vi "UHR-Fleezers Control (host) - 10.5.vi"() -> ()   [LabVIEW 2011] (continued)
        n935 = xnode "Read/Write Control"("FPGA VI Reference In"=w1438, "error in"=w1437, "Scan steps"=w1377, "Number of scans"="Number of F/B Scans (AOD)", "Cycles per step"=w1345, "Scan freq.  increment"=w1383, "Scan BD"="Scan BD") -> ("error out"=w1436:errorcluster)  [unwired: 1 out]
        n936 = Multiply(x=w1377, y=w1345) -> (x*y=w1431:u64)
        n937 = Multiply(x=w1431, y=u64 2) -> (x*y=w1353:u64)
        n938 = Multiply(x=w1354, y=w1353) -> (x*y=w1352:dbl)
        "Data points/scan (f/b)" <- w1352
        n939 = Multiply(x=w1352, y="Number of F/B Scans (AOD)") -> (x*y=w1434:dbl)
        "Data points/scans" <- w1434
        n940 = Divide(x=w1434, y=w1388) -> (x/y=→"N sets should be saved":dbl)
        n941 = Multiply(x=w1431, y=w1372) -> (x*y=w1370:dbl)
        "Time/Scan (s) (AOD)" <- w1370
        n942 = Select(t=w1402, s="Scan BD", f=0.0) -> (s? t:f=w1428:dbl)
        n943 = Select(t=0.0, s="Scan BD", f=w1402) -> (s? t:f=w1424:dbl)
        n944 = local read "BD 2 Frequency 2 (MHz)"() -> (w1420:dbl)
        n945 = local read "BD 1 Frequency 2 (MHz)"() -> (w1423:dbl)
        n946 = Add(x=w1424, y=w1395) -> (x+y=w1421:dbl)
        n947 = Add(x=w1389, y=w1428) -> (x+y=w1422:dbl)
        n948 = Multiply(x=w1370, y=2.0) -> (x*y=w1369:dbl)
        n949 = Multiply(x=w1369, y="Number of F/B Scans (AOD)") -> (x*y=w1366:dbl)
        n950 = Divide(x=w1366, y=60.0) -> (x/y=→"Time to Finish All (min)":dbl)
        n951 = Add(x="Trap 2 Bead Size (nm)", y="Trap 1 Bead Size (nm)") -> (x+y=w1410:dbl)
        n952 = Divide(x=w1410, y=2.0) -> (x/y=w1404:dbl)
        n953 = local read "Initial delta (MHz)"() -> (w1407:dbl)
        n954 = Subtract(x=w1421, y=w1420) -> (x-y=w1418:dbl)
        n955 = Subtract(x=w1422, y=w1423) -> (x-y=w1419:dbl)
        n956 = Square(x=w1418) -> (x^2=w1417:dbl)
        n957 = Square(x=w1419) -> (x^2=w1416:dbl)
        n958 = Add(x=w1416, y=w1417) -> (x+y=w1415:dbl)
        n959 = Square Root(x=w1415) -> (sqrt(x)=w1414:dbl)
        "Final delta (MHz)" <- w1414
        n960 = Multiply(x=w1406, y=w1414) -> (x*y=w1413:dbl)
        n961 = Multiply(x=w1407, y=w1406) -> (x*y=w1405:dbl)
        n962 = Subtract(x=w1405, y=w1404) -> (x-y=→"Initial sep (nm)":dbl)
        n963 = Subtract(x=w1413, y=w1404) -> (x-y=→"Final sep (nm)":dbl)
      }
      event "Freq or Amp switch first", "Swap F1 and F2", "Freq switch delay", "Amp switch delay": Value Change {
        n964 = event-data() -> ()  [unwired: 7 out]
        n965 = local read "Freq or Amp switch first"() -> (w1439:bool)
        n966 = local read "Amp switch delay"() -> (w1440:u16)
        n967 = local read "Freq switch delay"() -> (w1442:u16)
        n968 = local read "Swap F1 and F2"() -> (w1441:bool)
        n969 = xnode "Read/Write Control"("FPGA VI Reference In"=w1445, "error in"=w1444, "Freq switch delay"=w1442, "Swap F1 and F2"=w1441, "Amp switch delay"=w1440, "Freq or Amp switch first"=w1439) -> ("error out"=w1443:errorcluster)  [unwired: 1 out]
      }
      event "Scan steps (MCL)", "Number of scans (MCL)", "Scan Range (V)\n(of steps)", "2D or 1D Scan", "N APD Samp/step", "Fast Scan Dir", "Continuous MCL Scanning", "Scan lines (y)": Value Change {
        w1447 = 32767.0 ("y")
        n970 = event-data() -> ()  [unwired: 7 out]
        n971 = Select(t="Scan lines (y)", s="2D or 1D Scan", f="Number of scans (MCL)") -> (s? t:f=w1452:u64)
        n972 = Decrement(x="Scan steps (MCL)") -> (x-1=w1468:u64)
        n973 = Divide(x="Scan Range (V)\n(of steps)", y=w1468) -> (x/y=w1467:dbl)
        "Desired Scan Incr (V)" <- w1467
        n974 = local read "APD Integration Time (s)"() -> (w1460:dbl)
        n975 = Multiply(x=w1467, y=w1447) -> (x*y=w1476:dbl)
        n976 = Divide(x=w1476, y=10.0) -> (x/y=w1466:dbl)
        "Desired incr (int)" <- w1466
        n977 = local read "Update Count (MCL)"() -> (w1472:u32)
        n978 = Round Toward -Infinity(1:w1466) -> (0:w1475:dbl)
        n979 = To Word Integer(number=w1475) -> (16bit integer=w1450:i16)
        "Actual Incr. int (MCL)" <- w1450
        n980 = Multiply(x=w1460, y=40000000.0) -> (x*y=w1473:dbl)
        n981 = Divide(x=w1473, y=w1472) -> (x/y=w1471:dbl)
        n982 = Multiply(x=i16 10, y=w1450) -> (x*y=w1448:i16)
        n983 = Multiply(x="N APD Samp/step", y=w1471) -> (x*y=w1470:dbl)
        "Cycles/step (MCL)" <- w1470
        n984 = Divide(x=w1448, y=w1447) -> (x/y=→"Actual MCL Inc (V)":dbl)
        n985 = Multiply(x="N APD Samp/step", y="Scan steps (MCL)") -> (x*y=w1462:dbl)
        n986 = local read "APD Samples/FIFO Acq."() -> (w1459:dbl)
        n987 = Multiply(x=w1462, y=u64 2) -> (x*y=w1461:dbl)
        "Data points/scan (f+b)" <- w1461
        n988 = Multiply(x=w1461, y=w1452) -> (x*y=w1479:dbl)
        "Data points/scans (MCL)" <- w1479
        n989 = Multiply(x=w1460, y=w1461) -> (x*y=w1453:dbl)
        "Time/f+b scan (s) (MCL)" <- w1453
        n990 = Divide(x=w1479, y=w1459) -> (x/y=→"N sets should be saved (MCL)":dbl)
        n991 = Multiply(x=w1453, y=w1452) -> (x*y=→"Total Time (s)":dbl)
        n992 = Not(x="Fast Scan Dir") -> (.not. x?=w1457:bool)
        n993 = xnode "Read/Write Control"("FPGA VI Reference In"=w1483, "error in"=w1482, "Scan steps (MCL)"="Scan steps (MCL)", "Number of scans (MCL)"=w1452, "Cycles per step (MCL)"=w1470, "Scan freq.  increment (MCL)"=w1450, "1D or 2D Scan?"="2D or 1D Scan", "MCL Scan Axis"=w1457, "Cont. Scan (MCL)"="Continuous MCL Scanning") -> ("error out"=w1481:errorcluster)  [unwired: 1 out]
      }
      event "Read Cal": Value Change {
        w1485 = 1000.0 ("y")
        n994 = event-data() -> ()  [unwired: 7 out]
        n995 = local read "Save file name"() -> (w1510:path)
        n996 = local write "Read Cal"(FALSE ("Read Cal")) -> ()
        n997 = Strip Path(path=w1510) -> (stripped path=w1509:path)  [unwired: 1 out]
        n998 = Path To String(path=w1509) -> (string=w1508:string)
        n999 = Concatenate Strings(w1508, "\\current.cal" ("string")) -> (w1506:string)
        n1000 = String To Path(string=w1506) -> (path=w1505:path)
        n1001 = Open/Create/Replace File(file path (use dialog)=w1505, operation (0:open)=T25."open", access (0:read/write)=enum16{"read/write", "read-only", "write-only"}."read-only") -> (refnum out=w1513:refnum<file>, error out=w1499:errorcluster)  [unwired: 1 in, 3 out]
        n1002 = Deny Access(4:w1499, 7:w1513) -> (0:w1498:errorcluster, 3:w1504:refnum<file>)  [unwired: 1 out]
        n1003 = Read from Binary File(5:0.0, 8:w1498, 9:T24."big-endian, network order" ("byte order (0:big-endian, network order)"), 10:-1 ("count (1)"), 11:w1504) -> (0:w1497:errorcluster, 2:w1495:dbl[], 3:w1500:refnum<file>)  [unwired: 2 out]
        n1004 = Array To Cluster(array=w1495) -> (cluster=w1494:T27)
        n1005 = Unbundle(w1494) -> ("[0]"=w1493:dbl, "[1]"=w1492:dbl, "[2]"=w1491:dbl, "[3]"=w1490:dbl, "[4]"=w1489:dbl, "[5]"=w1488:dbl)
        n1006 = Close File(refnum=w1500, error in=w1497) -> (error out=→"Read cal error":errorcluster)  [unwired: 1 out]
        n1007 = Multiply(x=w1488, y=w1485) -> (x*y=w1486:dbl)
        n1008 = local write "T2 kappa_x (pN/nm)"(w1490) -> ()
        n1009 = local write "T1 kappa_x (pN/nm)"(w1491) -> ()
        n1010 = local write "T1 alpha_x (nm/V)"(w1493) -> ()
        n1011 = local write "T2 alpha_x (nm/V)"(w1492) -> ()
        n1012 = Multiply(x=w1489, y=w1485) -> (x*y=w1487:dbl)
        n1013 = local write "T1 offset_x (mV)"(w1487) -> ()
        n1014 = local write "T2 offset_x (mV)"(w1486) -> ()
      }
      event "Abort MCL Scan": Value Change {
        n1015 = event-data() -> ()  [unwired: 7 out]
        n1016 = local write "MCL Scanning"(FALSE ("MCL Scanning")) -> ()
        n1017 = xnode "Read/Write Control"("FPGA VI Reference In"=w1518, "error in"=w1517, "Abort scan (MCL)"="Abort MCL Scan") -> ("error out"=w1516:errorcluster)  [unwired: 1 out]
      }
      event "Update Count (MCL)": Value Change {
        n1018 = event-data() -> ()  [unwired: 7 out]
        n1019 = xnode "Read/Write Control"("FPGA VI Reference In"=w1522, "error in"=w1521, "MCL count"="Update Count (MCL)") -> ("error out"=w1520:errorcluster)  [unwired: 1 out]
      }
      event "Phase adjust (MCL)", "+ phase (MCL)", "- phase (MCL)": Value Change {
        n1020 = event-data() -> ()  [unwired: 7 out]
        n1021 = Negate(x="Phase adjust (MCL)") -> (-x=w1531:i16)
        n1022 = Select(t=w1531, s="- phase (MCL)", f="Phase adjust (MCL)") -> (s? t:f=w1529:i16)
        n1023 = Or(x="- phase (MCL)", y="+ phase (MCL)") -> (x .or. y?=w1524:bool)
        n1024 = xnode "Read/Write Control"("FPGA VI Reference In"=w1533, "error in"=w1532, "Phase count adjustment (MCL)"=w1529) -> ("FPGA VI Reference Out"=w1525:T19, "error out"=w1526:errorcluster)
        n1025 = xnode "Read/Write Control"("FPGA VI Reference In"=w1525, "error in"=w1526, "+ phase (MCL)"=w1524) -> ("error out"=w1523:errorcluster)  [unwired: 1 out]
      }
      event "Abort AOD Scan": Value Change {
        n1026 = event-data() -> ()  [unwired: 7 out]
        n1027 = xnode "Read/Write Control"("FPGA VI Reference In"=w1537, "error in"=w1536, "Abort scan"="Abort AOD Scan") -> ("error out"=w1535:errorcluster)  [unwired: 1 out]
      }
      event "Continuous AOD Scanning": Value Change {
        n1028 = event-data() -> ()  [unwired: 7 out]
        n1029 = xnode "Read/Write Control"("FPGA VI Reference In"=w1541, "error in"=w1540, "Cont. Scan"="Continuous AOD Scanning") -> ("error out"=w1539:errorcluster)  [unwired: 1 out]
      }
      event "Index": Value Change {
        n1030 = event-data() -> ()  [unwired: 7 out]
        n1031 = call "Create new save file.vi"("Insert"="", "Ext"=".dat" ("string"), "Index In"="Index") -> ("Path Out"=→"Save file name":path, "Index Out"=w1542:dbl)
        "Save index" <- w1542
        n1032 = local write "Index"(w1542) -> ()
      }
      event "AO1", "AO2": Value Change {
        w1557 = 10.0 ("y")
        w1556 = 32767.0 ("y")
        n1033 = event-data() -> ()  [unwired: 7 out]
        n1034 = local read "AO2"() -> (w1555:dbl)
        n1035 = local read "AO1"() -> (w1552:dbl)
        n1036 = Multiply(x=w1552, y=w1556) -> (x*y=w1551:dbl)
        n1037 = Multiply(x=w1555, y=w1556) -> (x*y=w1554:dbl)
        n1038 = Divide(x=w1551, y=w1557) -> (x/y=w1550:dbl)
        n1039 = Divide(x=w1554, y=w1557) -> (x/y=w1553:dbl)
        n1040 = To Word Integer(number=w1550) -> (16bit integer=w1558:i16)
        n1041 = To Word Integer(number=w1553) -> (16bit integer=w1559:i16)
        n1042 = xnode "Read/Write Control"("FPGA VI Reference In"=w1549, "error in"=w1548, "AO1"=w1558, "AO2"=w1559) -> ("error out"=w1547:errorcluster)  [unwired: 1 out]
      }
      event "Inject Pump 1": Value Change {
        n1043 = local read "Chemyx Syringe Pump Serial Port"() -> (w1560:refnum<visa-resource-name>)
        n1044 = event-data() -> ()  [unwired: 7 out]
        n1045 = local read "Pump write delay (ms)"() -> (w1561:dbl)
        n1046 = case shown="False" "Inject Pump 1" {
          tunnel: w1561 -> [w1568 w1582]
          tunnel: w1560 -> [w1565 w1581]
          frame False {
            n1047 = flat-sequence {
              tunnel: w1565 -> [w1569]
              tunnel: [w1569] -> w1566
              tunnel: w1568 -> [_]
              tunnel: [w1572] -> w1567
              tunnel: w1566 -> [w1572]
              tunnel: w1567 -> [w1573]
              tunnel: [w1573] -> w1563
              tunnel: [w1575] -> w1564
              tunnel: w1563 -> [w1575]
              tunnel: w1564 -> [w1577]
              frame #0 {
                n1048 = call "Write to pump.vi"("string"="enter pump1", "VISA resource name"=w1569) -> ()  [unwired: 1 out]
              }
              frame #1 {
                n1049 = Wait (ms)(milliseconds to wait="Pump pause delay (ms)") -> ()  [unwired: 1 out]
              }
              frame #2 {
                n1050 = call "Write to pump.vi"("string"="stop", "VISA resource name"=w1573) -> ()  [unwired: 1 out]
              }
              frame #3 {
                n1051 = Wait (ms)(milliseconds to wait=u32 500) -> ()  [unwired: 1 out]
              }
              frame #4 {
                n1052 = call "Write to pump.vi"("string"="stop", "VISA resource name"=w1577) -> ()  [unwired: 1 out]
              }
            }
          }
          frame True {
            n1053 = flat-sequence {
              tunnel: w1581 -> [w1591]
              tunnel: w1582 -> [w1586]
              tunnel: w1582 -> [w1593]
              tunnel: w1581 -> [w1594]
              tunnel: [w1594] -> w1579
              tunnel: [w1596] -> w1580
              tunnel: w1579 -> [w1596]
              tunnel: w1580 -> [w1598]
              frame #0 {
                n1054 = local read "All Pump Parameters"() -> (w1585:T1)
                n1055 = Unbundle By Name(w1585) -> ("Pump 1"=w1592:T28)
                n1056 = call "Set pump parameters.vi"("Pump write delay (ms)"=w1586, "Volume (uL)"="Ch 1 Inject Volume (uL)", "Rate (uL/h)"="Ch 1 Inject Rate (ul/h)", "Units"=4.0, "Pump #"=1.0, "Pump Parameters In"=w1592, "VISA resource name"=w1591) -> ("Pump Parameters Out"=w1584:T28)  [unwired: 3 in]
                n1057 = Bundle By Name(cluster=w1585, "Pump 1"=w1584) -> (w1583:T1)
                n1058 = local write "All Pump Parameters"(w1583) -> ()
              }
              frame #1 {
                n1059 = Wait (ms)(milliseconds to wait=w1593) -> ()  [unwired: 1 out]
              }
              frame #2 {
                n1060 = call "Write to pump.vi"("string"="start", "VISA resource name"=w1594) -> ()  [unwired: 1 out]
              }
              frame #3 {
                n1061 = Wait (ms)(milliseconds to wait=u32 500) -> ()  [unwired: 1 out]
              }
              frame #4 {
                n1062 = call "Write to pump.vi"("string"="start", "VISA resource name"=w1598) -> ()  [unwired: 1 out]
              }
            }
          }
        }
      }
      event "Inject Pump 3": Value Change {
        n1063 = event-data() -> ()  [unwired: 7 out]
        n1064 = local read "Pump write delay (ms)"() -> (w1601:dbl)
        n1065 = case shown="False" "Inject Pump 3" {
          tunnel: w1601 -> [w1608 w1622]
          tunnel: "Chemyx Syringe Pump Serial Port" -> [w1605 w1621]
          frame False {
            n1066 = flat-sequence {
              tunnel: w1605 -> [w1609]
              tunnel: [w1609] -> w1606
              tunnel: w1608 -> [_]
              tunnel: [w1612] -> w1607
              tunnel: w1606 -> [w1612]
              tunnel: w1607 -> [w1613]
              tunnel: [w1613] -> w1603
              tunnel: [w1615] -> w1604
              tunnel: w1603 -> [w1615]
              tunnel: w1604 -> [w1617]
              frame #0 {
                n1067 = call "Write to pump.vi"("string"="enter pump3", "VISA resource name"=w1609) -> ()  [unwired: 1 out]
              }
              frame #1 {
                n1068 = local read "Pump pause delay (ms)"() -> (w1611:u32)
                n1069 = Wait (ms)(milliseconds to wait=w1611) -> ()  [unwired: 1 out]
              }
              frame #2 {
                n1070 = call "Write to pump.vi"("string"="stop", "VISA resource name"=w1613) -> ()  [unwired: 1 out]
              }
              frame #3 {
                n1071 = Wait (ms)(milliseconds to wait=u32 0) -> ()  [unwired: 1 out]
              }
              frame #4 {
                n1072 = call "Write to pump.vi"("string"="stop", "VISA resource name"=w1617) -> ()  [unwired: 1 out]
              }
            }
          }
          frame True {
            n1073 = flat-sequence {
              tunnel: w1621 -> [w1631]
              tunnel: w1622 -> [w1626]
              tunnel: w1622 -> [w1633]
              tunnel: w1621 -> [w1634]
              tunnel: [w1634] -> w1619
              tunnel: [w1637] -> w1620
              tunnel: w1619 -> [w1637]
              tunnel: w1620 -> [w1638]
              frame #0 {
                n1074 = local read "All Pump Parameters"() -> (w1625:T1)
                n1075 = Unbundle By Name(w1625) -> ("Pump 3"=w1632:T28)
                n1076 = call "Set pump parameters.vi"("Pump write delay (ms)"=w1626, "Volume (uL)"="Ch 3 Inject Volume (uL)", "Rate (uL/h)"="Ch 3 Inject Rate (ul/h)", "Units"=4.0, "Pump #"=3.0, "Pump Parameters In"=w1632, "VISA resource name"=w1631) -> ("Pump Parameters Out"=w1624:T28)  [unwired: 3 in]
                n1077 = Bundle By Name(cluster=w1625, "Pump 3"=w1624) -> (w1623:T1)
                n1078 = local write "All Pump Parameters"(w1623) -> ()
              }
              frame #1 {
                n1079 = Wait (ms)(milliseconds to wait=w1633) -> ()  [unwired: 1 out]
              }
              frame #2 {
                n1080 = call "Write to pump.vi"("string"="start", "VISA resource name"=w1634) -> ()  [unwired: 1 out]
              }
              frame #3 {
                n1081 = Wait (ms)(milliseconds to wait=u32 500) -> ()  [unwired: 1 out]
              }
              frame #4 {
                n1082 = call "Write to pump.vi"("string"="start", "VISA resource name"=w1638) -> ()  [unwired: 1 out]
              }
            }
          }
        }
      }
      event "Inject Pump 2": Value Change {
        n1083 = event-data() -> ()  [unwired: 7 out]
        n1084 = local read "Pump write delay (ms)"() -> (w1642:dbl)
        n1085 = flat-sequence {
          tunnel: w1640 -> [w1655]
          tunnel: w1642 -> [w1651]
          tunnel: "Inject Pump 2" -> [_]
          tunnel: w1642 -> [w1657]
          tunnel: w1640 -> [w1658]
          frame #0 {
            n1086 = local read "All Pump Parameters"() -> (w1650:T1)
            n1087 = Multiply(x=60.0, y="Flush Center Ch Rate (ul/m)") -> (x*y=w1647:dbl)
            n1088 = Unbundle By Name(w1650) -> ("Pump 2"=w1656:T28)
            n1089 = call "Set pump parameters.vi"("Pump write delay (ms)"=w1651, "Volume (uL)"="Flush Center Ch Volume (uL)", "Rate (uL/h)"=w1647, "Units"=3.0, "Pump #"=2.0, "Pump Parameters In"=w1656, "VISA resource name"=w1655) -> ("Pump Parameters Out"=w1649:T28)  [unwired: 3 in]
            n1090 = Bundle By Name(cluster=w1650, "Pump 2"=w1649) -> (w1648:T1)
            n1091 = local write "All Pump Parameters"(w1648) -> ()
            n1092 = Add(x="Flush Center Ch Volume (uL)", y="Total Volume\nFlushed (uL)") -> (x+y=w1644:dbl)
            n1093 = local write "Total Volume\nFlushed (uL)"(w1644) -> ()
          }
          frame #1 {
            n1094 = Wait (ms)(milliseconds to wait=w1657) -> ()  [unwired: 1 out]
          }
          frame #2 {
            n1095 = call "Write to pump.vi"("string"="start", "VISA resource name"=w1658) -> ()  [unwired: 1 out]
          }
        }
        n1096 = local read "Chemyx Syringe Pump Serial Port"() -> (w1640:refnum<visa-resource-name>)
      }
      event "Sample Channel\nFlow": Value Change {
        n1097 = event-data() -> ()  [unwired: 7 out]
        n1098 = case shown="True" "Sample Channel\nFlow" {
          tunnel: w1662 -> [w1668 w1670]
          tunnel: [w1668 w1669] -> w1661
          frame False {
          }
          frame True {
            n1099 = Number To Decimal String(number="Flow rate (uL/h)") -> (decimal integer string=w1675:string)  [unwired: 1 in]
            n1100 = Concatenate Strings("irate  " ("string"), w1675, " u/h" ("string"), "\r") -> (w1673:string)
            n1101 = VISA Write(VISA resource name=w1670, write buffer=w1673) -> (VISA resource name out=w1669:refnum<visa-resource-name>)  [unwired: 1 in, 2 out]
          }
        }
        n1102 = Select(t="run" ("string"), s="Sample Channel\nFlow", f="stop" ("string")) -> (s? t:f=w1663:string)
        n1103 = Concatenate Strings(w1663, "\r") -> (w1666:string)
        n1104 = VISA Write(VISA resource name=w1661, write buffer=w1666) -> ()  [unwired: 1 in, 3 out]
      }
      event "Flow rate (uL/h)": Value Change {
        n1105 = event-data() -> ()  [unwired: 7 out]
        n1106 = local read "Flow rate (uL/h)"() -> (w1679:dbl)
        n1107 = Number To Decimal String(number=w1679) -> (decimal integer string=w1682:string)  [unwired: 1 in]
        n1108 = Concatenate Strings("irate  " ("string"), w1682, " u/h" ("string"), "\r") -> (w1681:string)
        n1109 = VISA Write(VISA resource name=w1677, write buffer=w1681) -> ()  [unwired: 1 in, 3 out]
      }
      event "Flush Sample": Value Change {
        n1110 = event-data() -> ()  [unwired: 7 out]
        n1111 = Number To Decimal String(number="Flush rate (uL/m)") -> (decimal integer string=w1701:string)  [unwired: 1 in]
        n1112 = Concatenate Strings("irate  " ("string"), w1701, " u/m" ("string"), "\r") -> (w1703:string)
        n1113 = VISA Write(VISA resource name=w1705, write buffer=w1703) -> (VISA resource name out=w1699:refnum<visa-resource-name>)  [unwired: 1 in, 2 out]
        n1114 = Number To Decimal String(number="Volume (uL)") -> (decimal integer string=w1688:string)  [unwired: 1 in]
        n1115 = Concatenate Strings("tvolume  " ("string"), w1688, " u" ("string"), "\r") -> (w1686:string)
        n1116 = VISA Write(VISA resource name=w1699, write buffer=w1686) -> (VISA resource name out=w1685:refnum<visa-resource-name>)  [unwired: 1 in, 2 out]
        n1117 = Concatenate Strings("cvolume" ("string"), "\r") -> (w1684:string)
        n1118 = VISA Write(VISA resource name=w1685, write buffer=w1684) -> (VISA resource name out=w1697:refnum<visa-resource-name>)  [unwired: 1 in, 2 out]
        n1119 = Concatenate Strings("run" ("string"), "\r") -> (w1695:string)
        n1120 = VISA Write(VISA resource name=w1697, write buffer=w1695) -> ()  [unwired: 1 in, 3 out]
      }
      event "Clear Volume": Value Change {
        n1121 = event-data() -> ()  [unwired: 7 out]
        n1122 = Concatenate Strings("cvolume" ("string"), "\r") -> (w1708:string)
        n1123 = VISA Write(VISA resource name=w1707, write buffer=w1708) -> ()  [unwired: 1 in, 3 out]
      }
      event "Flip Green Filter": Value Change {
        n1124 = event-data() -> ()  [unwired: 7 out]
        n1125 = Not(x="Flip Green Filter") -> (.not. x?=w1712:bool)
        n1126 = local write "Flip Green Filter"(w1712) -> ()
        n1127 = flat-sequence {
          tunnel: w1720 -> [w1725]
          tunnel: w1719 -> [w1724]
          tunnel: [w1722] -> w1717
          tunnel: [w1721] -> w1716
          tunnel: [w1727] -> w1715
          tunnel: w1717 -> [w1727]
          tunnel: [w1726] -> w1714
          tunnel: w1716 -> [w1726]
          tunnel: w1715 -> [w1731]
          tunnel: w1714 -> [w1730]
          tunnel: [w1729] -> w1718
          frame #0 {
            n1128 = xnode "Read/Write Control"("FPGA VI Reference In"=w1725, "error in"=w1724, "Green Filter Flipper"=TRUE) -> ("FPGA VI Reference Out"=w1722:T19, "error out"=w1721:errorcluster)
          }
          frame #1 {
            n1129 = Wait (ms)(milliseconds to wait=u32 100) -> ()  [unwired: 1 out]
          }
          frame #2 {
            n1130 = xnode "Read/Write Control"("FPGA VI Reference In"=w1731, "error in"=w1730, "Green Filter Flipper"=FALSE) -> ("error out"=w1729:errorcluster)  [unwired: 1 out]
          }
        }
      }
      event "Pump 1 contents", "Pump 3 contents": Value Change {
        n1131 = event-data() -> ()  [unwired: 7 out]
        n1132 = local read "Pump 1 contents"() -> (→"Pump 1 cont disp":string)
        n1133 = local read "Pump 3 contents"() -> (→"Pump 3 cont disp":string)
      }
      event "Reset Trap Pos. FB": Value Change {
        n1134 = event-data() -> ()  [unwired: 7 out]
        n1135 = xnode "Read/Write Control"("FPGA VI Reference In"=w1737, "error in"=w1736, "Trap Pos. FB Reset"="Reset Trap Pos. FB") -> ()  [unwired: 2 out]
      }
      event "Rem fb disp offset": Value Change {
        n1136 = event-data() -> ()  [unwired: 7 out]
        n1137 = local write "Rem fb disp offset"(FALSE ("Rem fb disp offset")) -> ()
        n1138 = local read "Mean T1 Position (nm)"() -> (w1739:dbl)
        n1139 = local read "FB Trap Pos Offset"() -> (w1740:dbl)
        n1140 = Subtract(x=w1740, y=w1739) -> (x-y=w1738:dbl)
        n1141 = local write "FB Trap Pos Offset"(w1738) -> ()
      }
      event "Threshold (nm)": Value Change {
        n1142 = event-data() -> ()  [unwired: 7 out]
        n1143 = flat-sequence {
          tunnel: w1744 -> [w1752]
          tunnel: w1743 -> [w1751]
          tunnel: [w1745] -> w1742
          tunnel: w1742 -> [w1758]
          frame #0 {
            n1144 = xnode "Read/Write Control"("FPGA VI Reference In"=w1752, "error in"=w1751) -> ("FPGA VI Reference Out"=w1748:T19, "error out"=w1747:errorcluster, "FPGA TTrig Thresh"=w1749:i64)
            n1145 = local read "Threshold stored (nm)"() -> (w1757:dbl)
            n1146 = local read "Threshold (nm)"() -> (w1745:dbl)
            n1147 = local read "AOM X Cal (nm/MHz)"() -> (w1755:dbl)
            n1148 = Subtract(x=w1745, y=w1757) -> (x-y=w1756:dbl)
            n1149 = Divide(x=w1756, y=w1755) -> (x/y=w1753:dbl)
            n1150 = call "IR AOM freq to word.vi"("Frequency In (MHz)"=w1753) -> ("Frequency Word Out (double)"=w1754:dbl)
            n1151 = To Quad Integer(1:w1754) -> (0:w1750:i64)
            n1152 = Add(x=w1749, y=w1750) -> (x+y=w1746:i64)
            n1153 = xnode "Read/Write Control"("FPGA VI Reference In"=w1748, "error in"=w1747, "FPGA TTrig Thresh"=w1746) -> ()  [unwired: 2 out]
          }
          frame #1 {
            "Threshold stored (nm)" <- w1758
          }
        }
      }
      event "FB Trig Integrate": Value Change {
        n1154 = event-data() -> ()  [unwired: 7 out]
        n1155 = local read "FB Trig Integrate"() -> (w1760:u32)
        n1156 = xnode "Read/Write Control"("FPGA VI Reference In"=w1762, "error in"=w1761, "FB Trig Integrate"=w1760) -> ("error out"=w1759:errorcluster)  [unwired: 1 out]
      }
      event "11": Value Change {
        n1157 = event-data() -> ()  [unwired: 7 out]
        n1158 = local read "11"() -> (w1763:bool)
        n1159 = case shown="True" w1763 {
          frame False {
          }
          frame True {
            n1160 = local read "Messages"() -> (w1765:string)
            n1161 = call "Update messages.vi"("Message to add"="You kicked it up to 11!", "Old message string"=w1765) -> ("New message string"=w1766:string)
            n1162 = call <vilib>:"Beep.vi"() -> ()  [unwired: 12 in]
            n1163 = local write "Messages"(w1766) -> ()
          }
        }
      }
      event "Trap Pos. FB ON": Value Change {
        n1164 = event-data() -> ()  [unwired: 7 out]
        n1165 = xnode "Read/Write Control"("FPGA VI Reference In"=w1769, "error in"=w1768, "Force feedback"="Trap Pos. FB ON") -> ()  [unwired: 2 out]
      }
      event "Remove Action Offset": Value Change {
        n1166 = event-data() -> ()  [unwired: 7 out]
        n1167 = local write "Remove Action Offset"(FALSE ("Remove Action Offset")) -> ()
        n1168 = local read "Trap Pos. FB Mult Factor"() -> (w1774:i64)
        n1169 = local read "Trap Pos FB Action"() -> (w1772:i64)
        n1170 = local read "Trap Pos. FB Offset Factor"() -> (w1770:i64)
        n1171 = Multiply(x=w1774, y=w1772) -> (x*y=w1773:i64)
        n1172 = Add(x=w1773, y=w1770) -> (x+y=w1771:i64)
        n1173 = local write "Trap Pos. FB Offset Factor"(w1771) -> ()
        n1174 = xnode "Read/Write Control"("FPGA VI Reference In"=w1777, "error in"=w1776, "Trap Pos. FB Offset Factor"=w1771) -> ()  [unwired: 2 out]
      }
      event "Remove Unwinding Offset": Value Change {
        n1175 = event-data() -> ()  [unwired: 7 out]
        n1176 = local write "Remove Unwinding Offset"(FALSE ("Remove Action Offset")) -> ()
        n1177 = local read "Trap Pos. FB Mult Factor"() -> (w1789:i64)
        n1178 = local read "Trap Pos FB Action"() -> (w1787:i64)
        n1179 = local read "Trap Pos. FB Offset Factor"() -> (w1786:i64)
        n1180 = Multiply(x=w1789, y=w1787) -> (x*y=w1788:i64)
        n1181 = local read "Trap Pos. FB Mult Factor"() -> (w1785:i64)
        n1182 = Add(x=w1788, y=w1786) -> (x+y=w1779:i64)
        n1183 = Multiply(x=32768, y="factor") -> (x*y=w1782:dbl)
        n1184 = Multiply(x=w1782, y=w1785) -> (x*y=w1784:dbl)
        n1185 = Subtract(x=w1779, y=w1784) -> (x-y=w1783:dbl)
        n1186 = To Quad Integer(1:w1783) -> (0:w1778:i64)
        n1187 = xnode "Read/Write Control"("FPGA VI Reference In"=w1792, "error in"=w1791, "Trap Pos. FB Offset Factor"=w1778) -> ()  [unwired: 2 out]
        n1188 = local write "Trap Pos. FB Offset Factor"(w1778) -> ()
      }
      event "Trap Pos. FB Range", "Trap Pos. FB Gains", "Trap Pos. FB Mult Factor", "Trap Pos. FB Offset Factor", "Trap Pos FB Negate Action", "Trap Pos FB Monitor\nT1 or T2", "Differential FB?", "Negate Diff?": Value Change {
        n1189 = event-data() -> ()  [unwired: 7 out]
        n1190 = local read "Negate Diff?"() -> (w1793:bool)
        n1191 = xnode "Read/Write Control"("FPGA VI Reference In"=w1803, "error in"=w1802, "Trap Pos. FB Range"="Trap Pos. FB Range", "Trap Pos. FB Gains"="Trap Pos. FB Gains", "Trap Pos. FB Mult Factor"="Trap Pos. FB Mult Factor", "Trap Pos. FB Offset Factor"="Trap Pos. FB Offset Factor", "Trap Pos FB Negate Action"="Trap Pos FB Negate Action", "Trap Pos FB Monitor T1 or T2"="Trap Pos FB Monitor\nT1 or T2", "AI1 X Scale"="Trap Pos. AI1 X Pre-scale", "Negate Diff?"=w1793, "Diff FB Measurement?"="Differential FB?") -> ()  [unwired: 2 out]
      }
      event "Trap Pos FB SP": Value Change {
        n1192 = event-data() -> ()  [unwired: 7 out]
        n1193 = xnode "Read/Write Control"("FPGA VI Reference In"=w1806, "error in"=w1805, "Trap Pos. FB SP"="Trap Pos FB SP") -> ()  [unwired: 2 out]
      }
      event "Set Reading to\nSetpoint": Value Change {
        # "This is the actual PID input signal"
        n1194 = event-data() -> ()  [unwired: 7 out]
        n1195 = local write "Set Reading to\nSetpoint"(FALSE ("Set SP to Reading")) -> ()
        n1196 = xnode "Read/Write Control"("FPGA VI Reference In"=w1811, "error in"=w1810) -> ("FPGA VI Reference Out"=w1809:T19, "error out"=w1808:errorcluster, "Trap Pos FB Int-Norm Signal"=w1807:fxp<+/-,16,1>)
        n1197 = local read "Differential FB?"() -> (w1812:bool)
        n1198 = case shown="False" w1812 {
          tunnel: [w1817 w1824] -> w1814
          tunnel: w1807 -> [w1815 w1824]
          frame False {
            n1199 = local read "Trap Pos FB Monitor\nT1 or T2"() -> (w1820:bool)
            n1200 = local read "Trap X AI1 (DMA)"() -> (w1823:T13)
            n1201 = Unbundle By Name(w1823) -> ("Set 1"=w1822:fxp<+/-,16,1>, "Set 2"=w1821:fxp<+/-,16,1>)
            n1202 = Select(t=w1822, s=w1820, f=w1821) -> (s? t:f=w1819:fxp<+/-,16,1>)
            n1203 = Not(x="Set SP Using...") -> (.not. x?=w1816:bool)
            n1204 = Select(t=w1815, s=w1816, f=w1819) -> (s? t:f=w1817:fxp<+/-,16,1>)
          }
          frame True {
          }
        }
        n1205 = xnode "Read/Write Control"("FPGA VI Reference In"=w1809, "error in"=w1808, "Trap Pos. FB SP"=w1814) -> ()  [unwired: 2 out]
        n1206 = local write "Trap Pos FB SP"(w1814) -> ()
      }
      event "Trap Pos. FB Out Scale 2^n": Value Change {
        n1207 = event-data() -> ()  [unwired: 7 out]
        n1208 = Scale By Power Of 2(n="Trap Pos. FB Out Scale 2^n", x=ext 1.0) -> (x*2^n=w1825:ext)
        n1209 = property on="Trap Pos. FB Mult Factor" class="DigNum (strict)"("Val(Sgnl)"=w1825) -> ()  [unwired: 2 in, 2 out]
      }
      event "Trap Pos FB Int Count": Value Change {
        n1210 = event-data() -> ()  [unwired: 7 out]
        n1211 = xnode "Read/Write Control"("FPGA VI Reference In"=w1830, "error in"=w1829, "Trap Pos FB Int Count"="Trap Pos FB Int Count") -> ()  [unwired: 2 out]
      }
    }
    "error out 2" <- w950
    n1212 = node-c288() -> ()  [unwired: 2 out]
  }
  n1213 = disable-structure shown="Disabled" {
    disable-tunnel: [w1832 _] -> w220
    disable-tunnel: w40 -> [w1831 _]
    frame Disabled {
      n1214 = node-c288() -> (w1834:T21)  [unwired: 4 out]
      n1215 = timed-loop "Rough control of MCL mirror stage (debugging)" {
        tunnel: w1831 -> [w1837]
        tunnel: [w1836] -> w1832
        timing: w1834 -> [_]
        timing-out: [_] -> w1833
        stop <- w1836 stop-if-true
        n1216 = node-c288() -> ()  [unwired: 2 out]
        n1217 = case shown="1" "MCL Mode" {
          tunnel: w1837 -> [_ w1840 w1887]
          frame 0, Default {
          }
          frame 1 {
            n1218 = node-c288() -> (w1842:T21)  [unwired: 4 out]
            n1219 = timed-loop "Oscillate MCL mirror" {
              timing: w1842 -> [_]
              timing-out: [_] -> w1841
              tunnel: w1840 -> [w1881]
              i -> [w1880]
              stop <- w1843 stop-if-true
              n1220 = node-c288() -> (w1879:i64)  [unwired: 1 out]
              n1221 = Multiply(x="AO1", y=32767.0) -> (x*y=w1875:dbl)
              n1222 = Multiply(x="AO2", y=32767.0) -> (x*y=w1870:dbl)
              n1223 = Divide(x=w1875, y=10.0) -> (x/y=w1876:dbl)
              n1224 = Divide(x=w1870, y=10.0) -> (x/y=w1871:dbl)
              n1225 = To Word Integer(number=w1876) -> (16bit integer=w1868:i16)
              n1226 = To Word Integer(number=w1871) -> (16bit integer=w1867:i16)
              n1227 = Divide(x=w1879, y=i64 1000) -> (x/y=w1850:dbl)
              n1228 = Multiply(x=w1850, y=w1880) -> (x*y=w1861:dbl)
              n1229 = Multiply(x="Osc. freq. (Hz) 2", y=6.283185307179586) -> (x*y=w1862:dbl)
              n1230 = Multiply(x=w1862, y=w1861) -> (x*y=w1860:dbl)
              n1231 = Sine(x=w1860) -> (sin(x)=w1859:dbl)
              n1232 = Multiply(x=w1859, y="Osc. amp. (V)") -> (x*y=w1857:dbl)
              n1233 = Add(x=w1857, y="Osc. center (V)") -> (x+y=w1855:dbl)
              n1234 = Divide(x=w1855, y=10.0) -> (x/y=w1853:dbl)
              n1235 = Multiply(x=w1853, y=32767.0) -> (x*y=w1848:dbl)
              n1236 = Select(t=w1848, s="Scan axis", f=w1868) -> (s? t:f=w1866:dbl)
              n1237 = Select(t=w1867, s="Scan axis", f=w1848) -> (s? t:f=w1865:dbl)
              n1238 = local read "MCL Mode"() -> (w1847:u16)
              n1239 = Not Equal?(x=w1847, y=u16 1) -> (x != y?=w1844:bool)
              n1240 = local read "Stop All"() -> (w1845:bool)
              n1241 = xnode "Read/Write Control"("FPGA VI Reference In"=w1881, "AO1"=w1866, "AO2"=w1865) -> ()  [unwired: 1 in, 2 out]
              n1242 = Compound Arithmetic op=OR(w1845, w1844) -> (w1843:bool)
              n1243 = node-c288() -> ()  [unwired: 2 out]
            }
            n1244 = node-c288(w1841) -> ()  [unwired: 1 out]
          }
          frame 2 {
            n1245 = case shown="True" "Start Scan" {
              tunnel: w1887 -> [_ w1899]
              frame False {
              }
              frame True {
                n1246 = Subtract(x="End (V)", y="Begin (V)") -> (x-y=w1895:dbl)
                n1247 = Decrement(x="N Points") -> (x-1=w1894:dbl)
                n1248 = Divide(x=w1895, y=w1894) -> (x/y=w1892:dbl)
                n1249 = for {
                  N: "N Points" -> [_]
                  tunnel: "Begin (V)" -> [w1912]
                  tunnel: w1899 -> [w1904]
                  tunnel: [w1903] -> w1898 mode=indexing
                  tunnel: w1892 -> [w1902]
                  tunnel: [w1900] -> w1891 mode=indexing
                  i -> [w1911]
                  n1250 = Multiply(x=w1902, y=w1911) -> (x*y=w1910:dbl)
                  n1251 = Add(x=w1912, y=w1910) -> (x+y=w1907:dbl)
                  n1252 = local read "Scan axis"() -> (w1901:bool)
                  n1253 = local read "AO1"() -> (w1909:dbl)
                  n1254 = local read "AO2"() -> (w1908:dbl)
                  n1255 = Select(t=w1907, s=w1901, f=w1909) -> (s? t:f=w1906:dbl)
                  n1256 = Select(t=w1908, s=w1901, f=w1907) -> (s? t:f=w1905:dbl)
                  n1257 = flat-sequence {
                    tunnel: w1906 -> [w1916]
                    tunnel: w1905 -> [w1915]
                    tunnel: w1904 -> [w1913]
                    tunnel: [w1926] -> w1903
                    tunnel: [w1925] -> w1900
                    frame #0 {
                      w1919 = 10.0 ("y")
                      w1914 = 32767.0 ("y")
                      n1258 = Multiply(x=w1916, y=w1914) -> (x*y=w1922:dbl)
                      n1259 = Multiply(x=w1915, y=w1914) -> (x*y=w1920:dbl)
                      n1260 = Divide(x=w1922, y=w1919) -> (x/y=w1923:dbl)
                      n1261 = Divide(x=w1920, y=w1919) -> (x/y=w1921:dbl)
                      n1262 = To Word Integer(number=w1923) -> (16bit integer=w1917:i16)
                      n1263 = To Word Integer(number=w1921) -> (16bit integer=w1918:i16)
                      n1264 = xnode "Read/Write Control"("FPGA VI Reference In"=w1913, "AO1"=w1917, "AO2"=w1918) -> ()  [unwired: 1 in, 2 out]
                    }
                    frame #1 {
                      n1265 = Wait (ms)(milliseconds to wait="DAQ Delay (ms)") -> ()  [unwired: 1 out]
                    }
                    frame #2 {
                      n1266 = local read "Slow mean"() -> (w1926:dbl)
                      n1267 = local read "Sigma"() -> (w1925:dbl)
                    }
                  }
                }
                n1268 = Bundle("Begin (V)"="Begin (V)", w1892, w1898) -> (→"MCL Scan":cluster{"Begin (V)":dbl, dbl, dbl[]})  [unwired: 1 out]
                n1269 = Bundle("Begin (V)"="Begin (V)", w1892, w1891) -> (→"MCL Scan 2":cluster{"Begin (V)":dbl, dbl, dbl[]})  [unwired: 1 out]
              }
            }
          }
        }
        n1270 = local read "Stop All"() -> (w1836:bool)
        n1271 = node-c288() -> ()  [unwired: 2 out]
      }
      n1272 = node-c288(w1833) -> ()  [unwired: 1 out]
    }
    frame Enabled {
    }
  }
  n1273 = node-c288() -> (w84:T21)  [unwired: 4 out]
  n1274 = node-c288(3 ("Processor")) -> (w80:T21)  [unwired: 3 out]
  n1275 = timed-loop "Mouse control: trap position (AOM deflection), set confocal spot from image" {
    tunnel: [w1930] -> w172
    tunnel: w40 -> [w1929]
    timing: w84 -> [_]
    timing-out: [_] -> w83
    stop <- w1930 stop-if-true
    n1276 = node-c288() -> ()  [unwired: 2 out]
    n1277 = event shown="[0] \"Pane\": Mouse Down" {
      selector: _ -> [_ _]
      dyn-events: _ -> [_ _]
      timeout: _ -> [_ _]
      tunnel: w1929 -> [w1933 _]
      event Mouse Down {
        n1278 = event-data() -> ("Time"=w1935:u32, "Coords"=w1934:T7, "Button"=w1936:u16)  [unwired: 6 out]
        n1279 = case shown="1" w1936 {
          tunnel: w1935 -> [_ _ w2039]
          tunnel: w1934 -> [_ w1973 w2037]
          tunnel: w1933 -> [_ _ w2035]
          frame 0, Default {
          }
          frame 1 {
            n1280 = property on="APD 2" class="ImageControl"() -> ("Displayed Image Position"=w1943:cluster{"Left":i32, "Top":i32})  [unwired: 2 in, 2 out]
            n1281 = property on="APD 1" class="ImageControl"() -> ("Displayed Image Position"=w1972:cluster{"Left":i32, "Top":i32})  [unwired: 2 in, 2 out]
            n1282 = property on="Detection Laser X" class="ImageControl"() -> ("Displayed Image Position"=w1969:cluster{"Left":i32, "Top":i32})  [unwired: 2 in, 2 out]
            n1283 = property on="Detection Laser Y" class="ImageControl"() -> ("Displayed Image Position"=w1968:cluster{"Left":i32, "Top":i32})  [unwired: 2 in, 2 out]
            n1284 = property on="APD 2" class="ImageControl"() -> ("Displayed Image Size"=w1942:cluster{"Width":u32, "Height":u32})  [unwired: 2 in, 2 out]
            n1285 = property on="APD 1" class="ImageControl"() -> ("Displayed Image Size"=w1970:cluster{"Width":u32, "Height":u32})  [unwired: 2 in, 2 out]
            n1286 = property on="Detection Laser X" class="ImageControl"() -> ("Displayed Image Size"=w1971:cluster{"Width":u32, "Height":u32})  [unwired: 2 in, 2 out]
            n1287 = property on="Detection Laser Y" class="ImageControl"() -> ("Displayed Image Size"=w1967:cluster{"Width":u32, "Height":u32})  [unwired: 2 in, 2 out]
            n1288 = Unbundle By Name(w1942) -> ("Width"=w1939:u32, "Height"=w1938:u32)
            n1289 = Unbundle By Name(w1943) -> ("Left"=w1941:i32, "Top"=w1940:i32)
            n1290 = Unbundle By Name(w1970) -> ("Width"=w1964:u32, "Height"=w1963:u32)
            n1291 = Unbundle By Name(w1971) -> ("Width"=w1960:u32, "Height"=w1959:u32)
            n1292 = Unbundle By Name(w1967) -> ("Width"=w1956:u32, "Height"=w1955:u32)
            n1293 = Unbundle By Name(w1972) -> ("Left"=w1966:i32, "Top"=w1965:i32)
            n1294 = Unbundle By Name(w1969) -> ("Left"=w1962:i32, "Top"=w1961:i32)
            n1295 = Unbundle By Name(w1968) -> ("Left"=w1958:i32, "Top"=w1957:i32)
            n1296 = Bundle("Left"=w1941, "Top"=w1940, "Width"=w1939, "Height"=w1938) -> (w1937:T29)  [unwired: 1 in]
            n1297 = Bundle("Left"=w1966, "Top"=w1965, "Width"=w1964, "Height"=w1963) -> (w1954:T29)  [unwired: 1 in]
            n1298 = Bundle("Left"=w1962, "Top"=w1961, "Width"=w1960, "Height"=w1959) -> (w1953:T29)  [unwired: 1 in]
            n1299 = Bundle("Left"=w1958, "Top"=w1957, "Width"=w1956, "Height"=w1955) -> (w1952:T29)  [unwired: 1 in]
            n1300 = Build Cluster Array(w1937, w1954, w1953, w1952) -> (w1951:T30)
            n1301 = for {
              tunnel: w1973 -> [w1984]
              tunnel: w1951 -> [w1985] mode=indexing
              shift-right: [w1982] -> w1949
              shift-left: TRUE -> [w1983]
              shift-right: [w1981] -> w1947
              shift-left: _ -> [w1977]
              shift-right: [w1980] -> w1946
              shift-left: _ -> [w1976]
              shift-right: [w1979] -> w1945
              shift-left: _ -> [w1975]
              shift-right: [w1978] -> w1944
              shift-left: _ -> [w1974]
              n1302 = case shown="True" w1983 {
                selector: w1983 -> [w1990 _]
                tunnel: w1985 -> [_ w1999]
                tunnel: w1984 -> [_ w1997]
                tunnel: [w1990 w1995] -> w1982
                tunnel: [w1989 w1994] -> w1981
                tunnel: [w1988 w1993] -> w1980
                tunnel: [w1987 w1992] -> w1979
                tunnel: [w1986 w1991] -> w1978
                tunnel: w1977 -> [w1989 _]
                tunnel: w1976 -> [w1988 _]
                tunnel: w1975 -> [w1987 _]
                tunnel: w1974 -> [w1986 _]
                frame False {
                }
                frame True {
                  n1303 = Unbundle(w1999) -> (w1998:T29)
                  n1304 = call "isclickinwindow.vi"("Image Param"=w1998, "Point32"=w1997) -> ("4 Y"=w1991:i32, "3 Height"=w1992:i32, "2 X"=w1993:i32, "1 Width"=w1994:i32, "In image?"=w1996:bool)  [unwired: 1 in]
                  n1305 = Not(x=w1996) -> (.not. x?=w1995:bool)
                }
              }
            }
            n1306 = Not(x=w1949) -> (.not. x?=w1948:bool)
            n1307 = case shown="True" w1948 {
              tunnel: w1946 -> [_ w2012]
              tunnel: w1944 -> [_ w2011]
              tunnel: w1947 -> [_ w2010]
              tunnel: w1945 -> [_ w2009]
              frame False {
              }
              frame True {
                w2005 = FALSE ("Get Point")
                n1308 = local read "Scan lines (y)"() -> (w2014:u64)
                n1309 = local read "Actual MCL Inc (V)"() -> (w2006:dbl)
                n1310 = local read "Scan steps (MCL)"() -> (w2013:u64)
                n1311 = Divide "Y Pix/step"(x=w2009, y=w2014) -> (x/y=w2021:dbl)
                n1312 = Divide "Y V/pix"(x=w2006, y=w2021) -> (x/y=w2020:dbl)
                n1313 = Divide "Y half step offset"(x=w2006, y=2.0) -> (x/y=w2022:dbl)
                n1314 = Divide "X pix/step"(x=w2010, y=w2013) -> (x/y=w2019:dbl)
                n1315 = Negate(x=w2022) -> (-x=w2023:dbl)
                n1316 = local read "Initial Y"() -> (w2029:dbl)
                n1317 = Multiply(x=w2011, y=w2020) -> (x*y=w2030:dbl)
                n1318 = Divide "X half step offset"(x=w2006, y=2.0) -> (x/y=w2016:dbl)
                n1319 = Divide "X V/pix"(x=w2006, y=w2019) -> (x/y=w2018:dbl)
                n1320 = Multiply(x=w2006, y=w2013) -> (x*y=w2025:dbl)
                n1321 = Compound Arithmetic op=ADD(w2023, w2030, w2029) -> (w2007:dbl)
                "Pointer Y (V)" <- w2007
                n1322 = Multiply(x=w2018, y=w2012) -> (x*y=w2027:dbl)
                n1323 = Negate(x=w2016) -> (-x=w2015:dbl)
                n1324 = local read "Initial X"() -> (w2028:dbl)
                n1325 = Negate(x=w2027) -> (-x=w2026:dbl)
                n1326 = Compound Arithmetic op=ADD(w2015, w2025, w2028, w2026) -> (w2008:dbl)
                "Pointer X (V)" <- w2008
                n1327 = Or(x="Set X Only", y="Set Confocal Spot (X-Y)") -> (x .or. y?=w2001:bool)
                n1328 = Or(x="Set Confocal Spot (X-Y)", y="Set Y Only") -> (x .or. y?=w2000:bool)
                n1329 = case shown="True" w2001 {
                  tunnel: w2008 -> [_ w2031]
                  frame False {
                  }
                  frame True {
                    n1330 = property on="AO2" class="Slide (strict)"("Val(Sgnl)"=w2031) -> ()  [unwired: 2 in, 2 out]
                  }
                }
                n1331 = case shown="True" w2000 {
                  tunnel: w2007 -> [_ w2032]
                  frame False {
                  }
                  frame True {
                    n1332 = property on="AO1" class="Slide (strict)"("Val(Sgnl)"=w2032) -> ()  [unwired: 2 in, 2 out]
                  }
                }
                n1333 = local write "Set Confocal Spot (X-Y)"(w2005) -> ()
                n1334 = local write "Set X Only"(w2005) -> ()
                n1335 = local write "Set Y Only"(w2005) -> ()
              }
            }
          }
          frame 3 {
            n1336 = local read "BD 2 Frequency 1 (MHz)"() -> (w2033:dbl)
            n1337 = local read "BD 1 Frequency 1 (MHz)"() -> (w2034:dbl)
            n1338 = local write "Manipulating Trap"(TRUE ("Manipulating Trap")) -> ()
            n1339 = local write "Coords"(T7 {"Horizontal"=0, "Vertical"=0} ("Coords")) -> ()
            n1340 = while {
              tunnel: w2039 -> [w2044]
              tunnel: w2037 -> [w2043]
              tunnel: w2035 -> [w2042]
              tunnel: w2034 -> [w2041]
              tunnel: w2033 -> [w2040]
              stop <- w2045 stop-if-true
              n1341 = event shown="[0] \"Pane\": Mouse Move" {
                selector: _ -> [_ _]
                dyn-events: _ -> [_ _]
                timeout: _ -> [_ _]
                tunnel: ["Force Manip Abort" w2109] -> w2045
                tunnel: w2044 -> [w2052 _]
                tunnel: w2043 -> [w2050 _]
                tunnel: w2042 -> [w2049 _]
                tunnel: w2041 -> [w2048 _]
                tunnel: w2040 -> [w2047 _]
                event Mouse Move {
                  n1342 = event-data() -> ("Time"=w2053:u32, "Coords"=w2054:T7)  [unwired: 3 out]
                  n1343 = Less?(x=w2053, y=w2052) -> (x < y?=w2051:bool)
                  n1344 = case "Makes sure old motion events prior to mouse click aren't used" shown="False" w2051 {
                    tunnel: w2054 -> [w2096 _]
                    tunnel: w2050 -> [w2097 _]
                    tunnel: w2049 -> [w2074 _]
                    tunnel: w2048 -> [w2070 _]
                    tunnel: w2047 -> [w2069 _]
                    frame False {
                      n1345 = Subtract(x=w2096, y=w2097) -> (x-y=w2095:T7)
                      "Coords" <- w2095
                      n1346 = local read "Y RF Frequency Limits (MHz)"() -> (w2055:T16)
                      n1347 = To Double Precision Float(number=w2095) -> (double precision float=w2094:cluster{"Horizontal":dbl, "Vertical":dbl})
                      n1348 = Multiply(x=cluster{"Horizontal":dbl, "Vertical":dbl} {"Horizontal"=-1.0, "Vertical"=1.0}, y="Manipulation Scaling") -> (x*y=w2090:cluster{"Horizontal":dbl, "Vertical":dbl})
                      n1349 = local read "X RF Frequency Limits (MHz)"() -> (w2056:T16)
                      n1350 = Multiply(x=w2094, y=w2090) -> (x*y=w2092:cluster{"Horizontal":dbl, "Vertical":dbl})
                      n1351 = Unbundle By Name(w2092) -> ("Horizontal"=w2087:dbl, "Vertical"=w2091:dbl)
                      n1352 = Unbundle By Name(w2055) -> ("Maximum"=w2058:dbl, "Minimum"=w2057:dbl)
                      n1353 = Boolean To (0,1)(Boolean="Manip. X?") -> (0, 1=w2085:i16)
                      n1354 = Boolean To (0,1)(Boolean="Manip. Y?") -> (0, 1=w2082:i16)
                      n1355 = local read "BD 1 Frequency 2 (MHz)"() -> (w2072:dbl)
                      n1356 = Multiply(x=w2091, y=w2082) -> (x*y=w2084:dbl)
                      n1357 = Multiply(x=w2085, y=w2087) -> (x*y=w2088:dbl)
                      n1358 = local read "BD 2 Frequency 2 (MHz)"() -> (w2071:dbl)
                      n1359 = Unbundle By Name(w2056) -> ("Maximum"=w2060:dbl, "Minimum"=w2059:dbl)
                      n1360 = Add(x=w2069, y=w2084) -> (x+y=w2062:dbl)
                      n1361 = Add(x=w2070, y=w2088) -> (x+y=w2064:dbl)
                      n1362 = In Range and Coerce(upper limit=w2060, x=w2064, lower limit=w2059) -> (coerced(x)=w2063:dbl)  [unwired: 1 out]
                      n1363 = In Range and Coerce(upper limit=w2058, x=w2062, lower limit=w2057) -> (coerced(x)=w2061:dbl)  [unwired: 1 out]
                      n1364 = Subtract(x=w2063, y=w2072) -> (x-y=w2081:dbl)
                      n1365 = Subtract(x=w2061, y=w2071) -> (x-y=w2080:dbl)
                      n1366 = Square(x=w2081) -> (x^2=w2079:dbl)
                      n1367 = Square(x=w2080) -> (x^2=w2078:dbl)
                      n1368 = Add(x=w2079, y=w2078) -> (x+y=w2077:dbl)
                      n1369 = Square Root(x=w2077) -> (sqrt(x)=w2073:dbl)
                      n1370 = In Range and Coerce(upper limit="Limit Max (MHz)", x=w2073, lower limit="Limit Min (MHz)") -> (In Range?=w2066:bool)  [unwired: 1 out]
                      n1371 = Not(x="Limits Enable") -> (.not. x?=w2065:bool)
                      n1372 = Or(x=w2066, y=w2065) -> (x .or. y?=w2067:bool)
                      n1373 = case shown="True" w2067 {
                        tunnel: w2074 -> [_ w2107]
                        tunnel: w2073 -> [_ w2098]
                        tunnel: w2063 -> [_ w2105]
                        tunnel: w2072 -> [_ w2104]
                        tunnel: w2061 -> [_ w2103]
                        tunnel: w2071 -> [_ w2102]
                        tunnel: w2056 -> [_ w2100]
                        tunnel: w2055 -> [_ w2099]
                        frame False {
                        }
                        frame True {
                          n1374 = local read "BD 1 Frequency 3 (MHz)"() -> (w2106:dbl)
